vi "Read Exception Status.vi"(8 "error in (no error)":errorcluster, 11 "MB session in":refnum<class "MB_Master.lvclass">) -> (0 "error out":errorcluster, 2 "Exception Status":u8 format="%.0x", 3 "MB session out":refnum<class "MB_Master.lvclass">)   [LabVIEW 2023, in "MB Master.lvlib"]
doc: "Function Code 7: Reads slave exception status"
uses:
  <vilib>/Plasmionique/MB Master/MB Master.lvlib
  <vilib>/Plasmionique/MB Master/MB_Master/MB_Master.lvclass
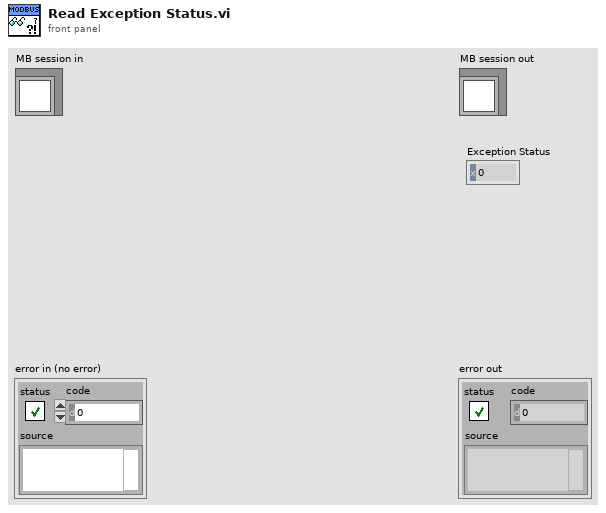
[diagram p1: front panel]
types:
  T1 = typedef "MB Master.lvlib/MB_PDU_Cluster.ctl" = cluster{"Function Code":u8, "Data":u8[], "RTU_DataBytes":i32}
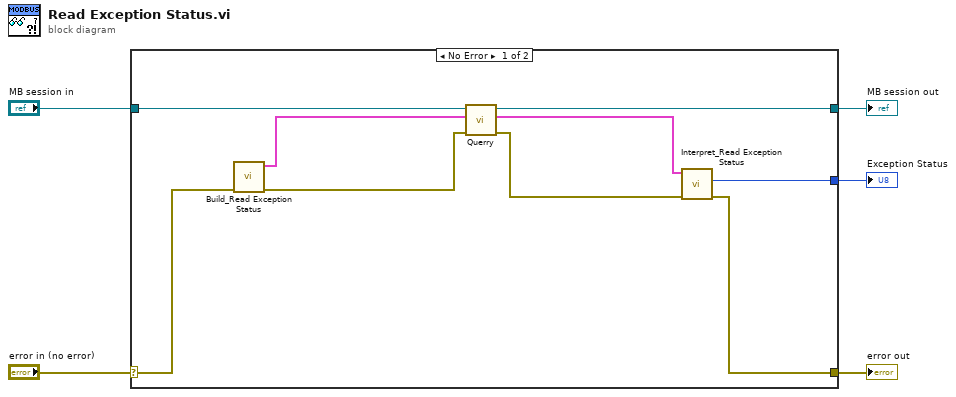
[diagram p0: block diagram]
diagram:
  n1 = case shown="No Error" "error in (no error)" {
    selector: "error in (no error)" -> [w12 w16]
    tunnel: [w11 w16] -> w4
    tunnel: [w7 w15] -> w2
    tunnel: "MB session in" -> [w10 w15]
    tunnel: [w6 _] -> w1
    frame No Error {
      n2 = call "Build_Read Exception Status.vi"("error in (no error)"=w12) -> ("error out"=w13:errorcluster, "MB_PDU"=w9:T1)  [unwired: 9 in]
      n3 = call-dynamic "Querry.vi"("error in (no error)"=w13, "PDU_req"=w9, "MB_Master in"=w10) -> ("error out"=w14:errorcluster, "PDU_resp"=w8:T1, "MB_Master out"=w7:refnum<class "MB_Master.lvclass">)  [unwired: 6 in]
      n4 = call "Interpret_Read Exception Status.vi"("error in (no error)"=w14, "MB_PDU_resp in"=w8) -> ("error out"=w11:errorcluster, "Exception Status"=w6:u8)  [unwired: 8 in]
    }
    frame Error {
    }
  }
  "error out" <- w4
  "MB session out" <- w2
  "Exception Status" <- w1
